vi "Write to Text Log File (Waveform).vi"(6 "Waveform Data":waveform(dbl)[](array[waveform]), 8 "error in (no error)":errorcluster, 9 "Channel Names in":string[](array[string]), 10 "Group Names in":string[](array[string]), 11 "Text Log File in":refnum<class "Text Log File.lvclass">) -> (0 "error out":errorcluster, 3 "Text Log File out":refnum<class "Text Log File.lvclass">)   [LabVIEW 2015, in "Text Log File.lvclass"]
uses:
  Text Log File.lvclass
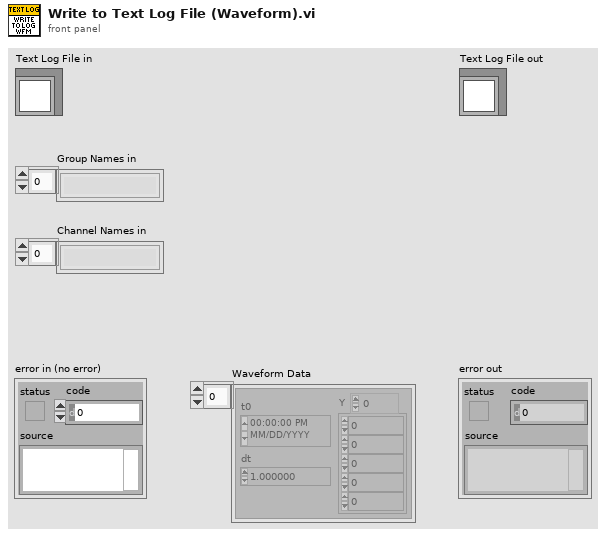
[diagram p1: front panel]
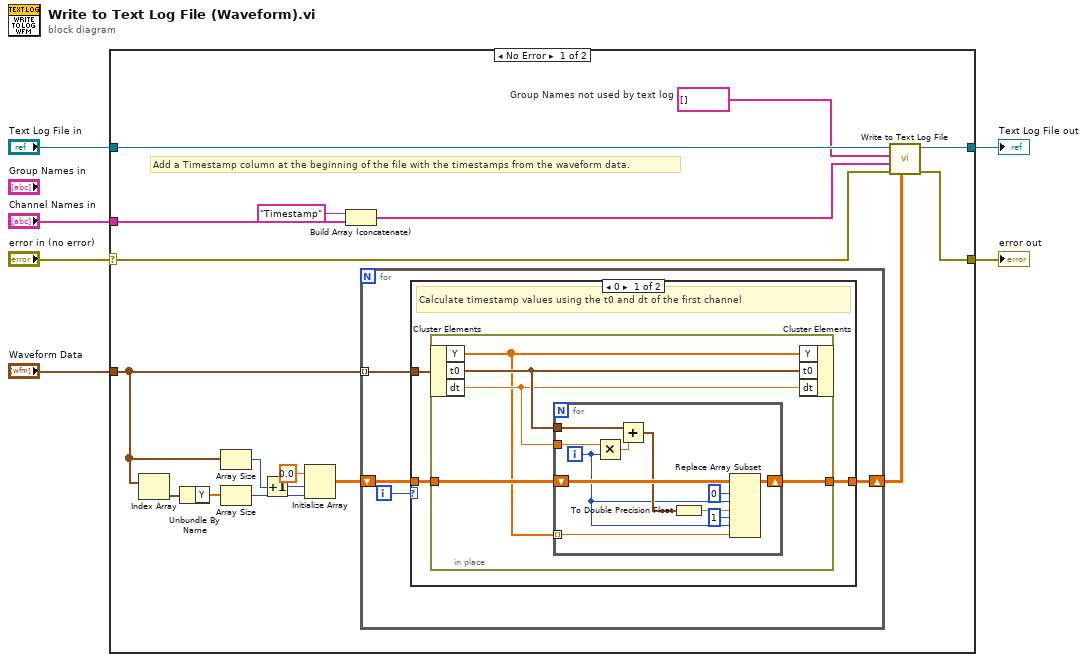
[diagram p0: block diagram]
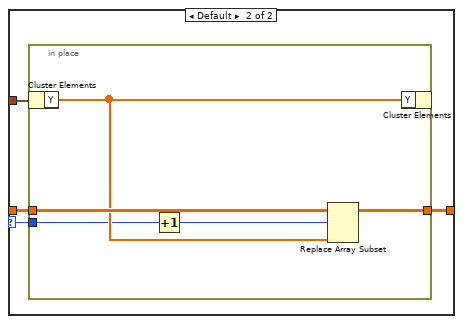
[diagram p2: hidden frame]
diagram:
  n1 = case shown="No Error" "error in (no error)" {
    selector: "error in (no error)" -> [w7 w57]
    tunnel: "Waveform Data" -> [w19 _]
    tunnel: "Text Log File in" -> [w15 w56]
    tunnel: [w14 w56] -> w4
    tunnel: "Channel Names in" -> [w13 _]
    tunnel: [w8 w57] -> w2
    frame No Error {
      w11 = string[] []  # Group Names not used by text log
      # "Add a Timestamp column at the beginning of the file with the timestamps from the waveform data."
      n2 = Index Array(array=w19) -> (element=w21:waveform(dbl))  [unwired: 1 in]
      n3 = Unbundle By Name(w21) -> ("Y"=w22:dbl[])
      n4 = Array Size(array=w19) -> (size(s)=w18:i32)
      n5 = Array Size(array=w22) -> (size(s)=w20:i32)
      n6 = Increment(x=w18) -> (x+1=w16:i32)
      n7 = Initialize Array(0.0, w16, w20) -> (w17:dbl[][])
      n8 = Build Array (concatenate)("Timestamp", w13) -> (w10:string[])
      n9 = for {
        tunnel: w19 -> [w26] mode=indexing
        shift-right: [w24] -> w9
        shift-left: w17 -> [w25]
        i -> [w27]
        n10 = case shown="0" w27 {
          selector: w27 -> [_ w47]
          tunnel: w26 -> [w30 w50]
          tunnel: w25 -> [w29 w49]
          tunnel: [w28 w48] -> w24
          frame 0 {
            # "Calculate timestamp values using the t0 and dt of the first channel"
            n11 = in-place {
              in-place-border: w29 -> [w33]
              in-place-border: [w32] -> w28
              n12 = in-place-cluster #1(w30) -> ("Y"=w31:dbl[], "t0"=w35:timestamp, "dt"=w34:dbl)
              n13 = for {
                tunnel: w35 -> [w45]
                tunnel: w34 -> [w46]
                shift-right: [w41] -> w32
                shift-left: w33 -> [w43]
                tunnel: w31 -> [w38] mode=indexing
                i -> [w36]
                n14 = Multiply(x=w46, y=w36) -> (x*y=w44:dbl)
                n15 = Add(x=w45, y=w44) -> (x+y=w39:timestamp)
                n16 = To Double Precision Float(number=w39) -> (double precision float=w40:dbl)
                n17 = Replace Array Subset(array=w43, new element #1=w40, index (row) #1=0 ("disabled index (row)"), index (col) #1=w36, new element #2=w38, index (row) #2=1 ("index (row)"), index (col) #2=w36) -> (w41:dbl[][])
              }
              n18 = in-place-cluster #1("Y"=w31, "t0"=w35, "dt"=w34) -> ()  [unwired: 1 out]
            }
          }
          frame Default {
            n19 = in-place {
              in-place-border: w49 -> [w55]
              in-place-border: [w54] -> w48
              in-place-border: w47 -> [w52]
              n20 = in-place-cluster #2(w50) -> ("Y"=w53:dbl[])
              n21 = Increment(x=w52) -> (x+1=w51:i32)
              n22 = Replace Array Subset(array=w55, new element=w53, index (row)=w51) -> (w54:dbl[][])  [unwired: 1 in]
              n23 = in-place-cluster #2("Y"=w53) -> ()  [unwired: 1 out]
            }
          }
        }
      }
      n24 = call "Write to Text Log File.vi"("Data"=w9, "error in (no error)"=w7, "Channel Names in"=w10, "Group Names in"=w11, "Text Log File in"=w15) -> ("error out"=w8:errorcluster, "Text Log File out"=w14:refnum<class "Text Log File.lvclass">)  [unwired: 5 in]
    }
    frame Error {
    }
  }
  "error out" <- w2
  "Text Log File out" <- w4
